vi "Delete_Last_Comma.vi"(11 "String":string) -> (3 "String 2":string)   [LabVIEW 2019, in "DAQ970.lvlib" / "DAQ970.lvclass"]
uses:
  Library/DAQ970.lvclass
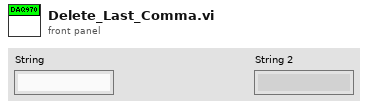
[diagram p1: front panel]
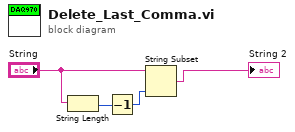
[diagram p0: block diagram]
diagram:
  n1 = String Length(string="String") -> (length=w3:i32)
  n2 = Decrement(x=w3) -> (x-1=w2:i32)
  n3 = String Subset(string="String", length (rest)=w2) -> (substring=→"String 2":string)  [unwired: 1 in]
